vi "PiShutdown.vi"   [LabVIEW 2013]
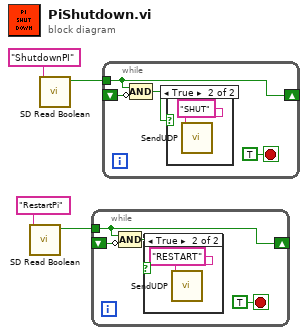
[diagram p0: block diagram]
diagram:
  n1 = call <vilib>:"SD Read Boolean.vi"("Name"="RestartPi") -> ("Boolean"=w2:bool)  [unwired: 8 in, 2 out]
  n2 = call <vilib>:"SD Read Boolean.vi"("Name"="ShutdownPI") -> ("Boolean"=w4:bool)  [unwired: 8 in, 2 out]
  n3 = while {
    tunnel: w2 -> [w7]
    shift-right: [w7] -> _
    shift-left: _ -> [w6]
    stop <- TRUE stop-if-true
    n4 = Compound Arithmetic op=AND(w7, invert w6) -> (w5:bool)
    n5 = case shown="True" w5 {
      frame False {
      }
      frame True {
        n6 = call "SendUDP.vi"("data in"="RESTART") -> ()  [unwired: 10 in, 1 out]
      }
    }
  }
  n7 = while {
    tunnel: w4 -> [w12]
    shift-right: [w12] -> _
    shift-left: _ -> [w11]
    stop <- TRUE stop-if-true
    n8 = Compound Arithmetic op=AND(w12, invert w11) -> (w10:bool)
    n9 = case shown="True" w10 {
      frame False {
      }
      frame True {
        n10 = call "SendUDP.vi"("data in"="SHUT") -> ()  [unwired: 10 in, 1 out]
      }
    }
  }
